vi "0~1随机数发生器（dbl).vi"(8 "Error In":errorcluster caption="错误输入") -> (0 "Error Out":errorcluster caption="错误输出", 3 "Rand(0-1)":dbl)   [LabVIEW 2013]
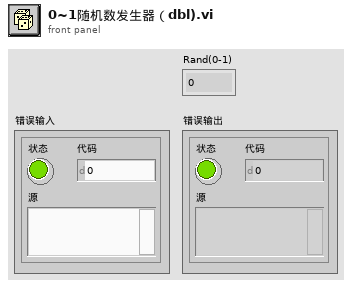
[diagram p1: front panel]
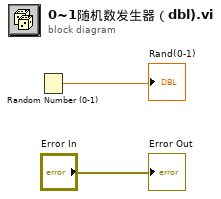
[diagram p0: block diagram]
diagram:
  n1 = Random Number (0-1)() -> (number: 0 to 1=→"Rand(0-1)":dbl)
  "Error Out" <- "Error In"
